vi "Read ID.vi"(8 "error in (no error)":errorcluster, 11 "Multimeter in":refnum<class "Multimeter.lvclass">) -> (0 "error out":errorcluster, 3 "Multimeter out":refnum<class "Multimeter.lvclass">)   [LabVIEW 2015, in "Multimeter.lvclass"]
doc: "VI used to Read Hardware ID"
uses:
  Multimeter.lvclass
  <instrlib>/Agilent 34401/Agilent 34401.lvlib
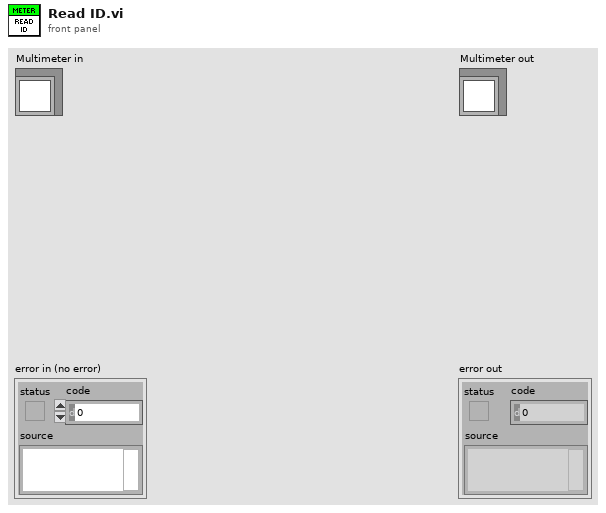
[diagram p1: front panel]
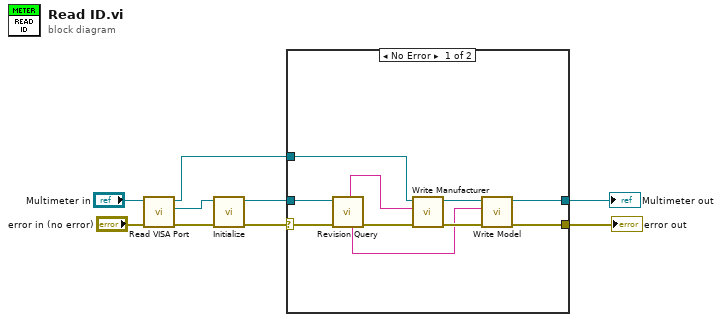
[diagram p0: block diagram]
diagram:
  n1 = call-dynamic "Read VISA Port.vi"("error in (no error)"="error in (no error)", "Device in"="Multimeter in") -> ("error out"=w6:errorcluster, "VISA Port"=w7:refnum<visa-resource-name>, "Device out"=w1:refnum<class "Multimeter.lvclass">)  [unwired: 7 in]
  n2 = call <instrlib>:"Initialize.vi"("error in (no error)"=w6, "VISA resource name"=w7) -> ("error out"=w2:errorcluster, "VISA resource name out"=w5:refnum<visa-resource-name>)  [unwired: 8 in]
  n3 = case shown="No Error" w2 {
    selector: w2 -> [w10 w20]
    tunnel: w5 -> [w19 _]
    tunnel: w1 -> [w18 w21]
    tunnel: [w12 w20] -> w4
    tunnel: [w11 w21] -> w3
    frame No Error {
      n4 = call <instrlib>:"Revision Query.vi"("error in (no error)"=w10, "VISA resource name"=w19) -> ("error out"=w16:errorcluster, "Modelo"=w13:string, "Fabricante"=w17:string)  [unwired: 4 in, 3 out]
      n5 = call-dynamic "Write Manufacturer.vi"("error in (no error)"=w16, "Manufacturer"=w17, "Device in"=w18) -> ("error out"=w15:errorcluster, "Device out"=w14:refnum<class "Multimeter.lvclass">)  [unwired: 7 in]
      n6 = call-dynamic "Write Model.vi"("error in (no error)"=w15, "Model"=w13, "Device in"=w14) -> ("error out"=w12:errorcluster, "Device out"=w11:refnum<class "Multimeter.lvclass">)  [unwired: 7 in]
    }
    frame Error {
    }
  }
  "error out" <- w4
  "Multimeter out" <- w3
